vi "JSONinst-GeneralProcessNames.vi"(8 "error in (no error)":errorcluster, 11 "ERP-CreateInstructions in":refnum<class "ERP-CreateInstructions.lvclass">) -> (0 "error out":errorcluster, 3 "ERP-CreateInstructions out":refnum<class "ERP-CreateInstructions.lvclass">, 5 "JSON string General InstData":string)   [LabVIEW 2013, in "ERP-CreateInstructions.lvclass"]
uses:
  ERP-CreateInstructions.lvclass
  ERP-CreateInstructions.lvclass/ERP-CreateInstructions.ctl
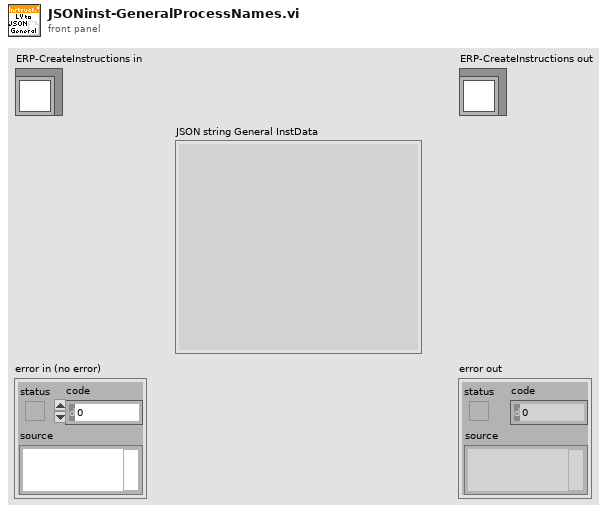
[diagram p1: front panel]
types:
  T1 = cluster{"General Process Step 1":string, "General Process Step 2":string, "General Process Step 3":string, "General Process Step 4":string, "General Process Step 5":string, "General Process Step 6":string}
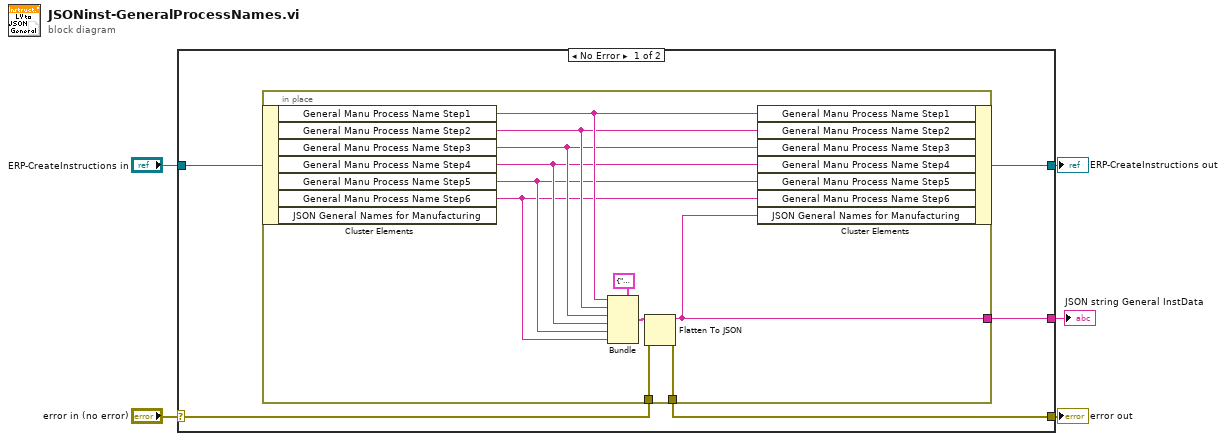
[diagram p0: block diagram]
diagram:
  n1 = case shown="No Error" "error in (no error)" {
    selector: "error in (no error)" -> [w10 w23]
    tunnel: [w9 w23] -> w4
    tunnel: [w7 w22] -> w2
    tunnel: "ERP-CreateInstructions in" -> [w8 w22]
    tunnel: [w6 _] -> w1
    frame No Error {
      n2 = in-place {
        in-place-border: w10 -> [w21]
        in-place-border: [w20] -> w9
        in-place-border: [w11] -> w6
        n3 = in-place-cluster #1(w8) -> ("General Manu Process Name Step1"=w17:string, "General Manu Process Name Step2"=w16:string, "General Manu Process Name Step3"=w15:string, "General Manu Process Name Step4"=w14:string, "General Manu Process Name Step5"=w13:string, "General Manu Process Name Step6"=w12:string)  [unwired: 1 out]
        n4 = Bundle(cluster=T1 {"General Process Step 1"="", "General Process Step 2"="", "General Process Step 3"="", "General Process Step 4"="", "General Process Step 5"="", "General Process Step 6"=""}, "General Process Step 1"=w17, "General Process Step 2"=w16, "General Process Step 3"=w15, "General Process Step 4"=w14, "General Process Step 5"=w13, "General Process Step 6"=w12) -> (w18:T1)
        n5 = Flatten To JSON(anything=w18, error in (no error)=w21) -> (JSON string=w11:string, 11:w20:errorcluster)  [unwired: 1 in]
        n6 = in-place-cluster #1("General Manu Process Name Step1"=w17, "General Manu Process Name Step2"=w16, "General Manu Process Name Step3"=w15, "General Manu Process Name Step4"=w14, "General Manu Process Name Step5"=w13, "General Manu Process Name Step6"=w12, "JSON General Names for Manufacturing"=w11) -> (w7:refnum<class "ERP-CreateInstructions.lvclass">)
      }
    }
    frame Error {
    }
  }
  "error out" <- w4
  "ERP-CreateInstructions out" <- w2
  "JSON string General InstData" <- w1
